vi "peakFinding dataSmooth.vi"(5 "Window":dbl=1.0 min=1.0 max=100000.0, 7 "Type":u8=1 min=1, 10 "dt":dbl=1.0, 11 "rawData":cluster{"xData":dbl[], "yData":dbl[]}) -> (3 "yData":dbl[](array[numeric]))   [LabVIEW 2018]
uses:
  PublicSubVI/Class/Sig2MS/Sig2MS.lvclass
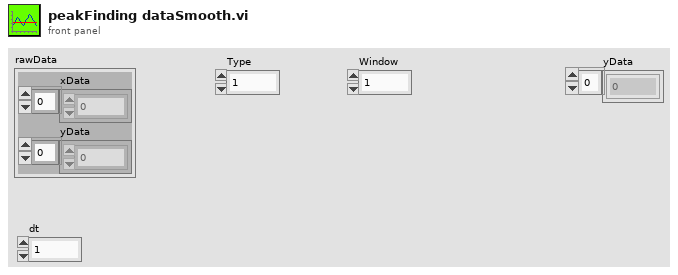
[diagram p1: front panel]
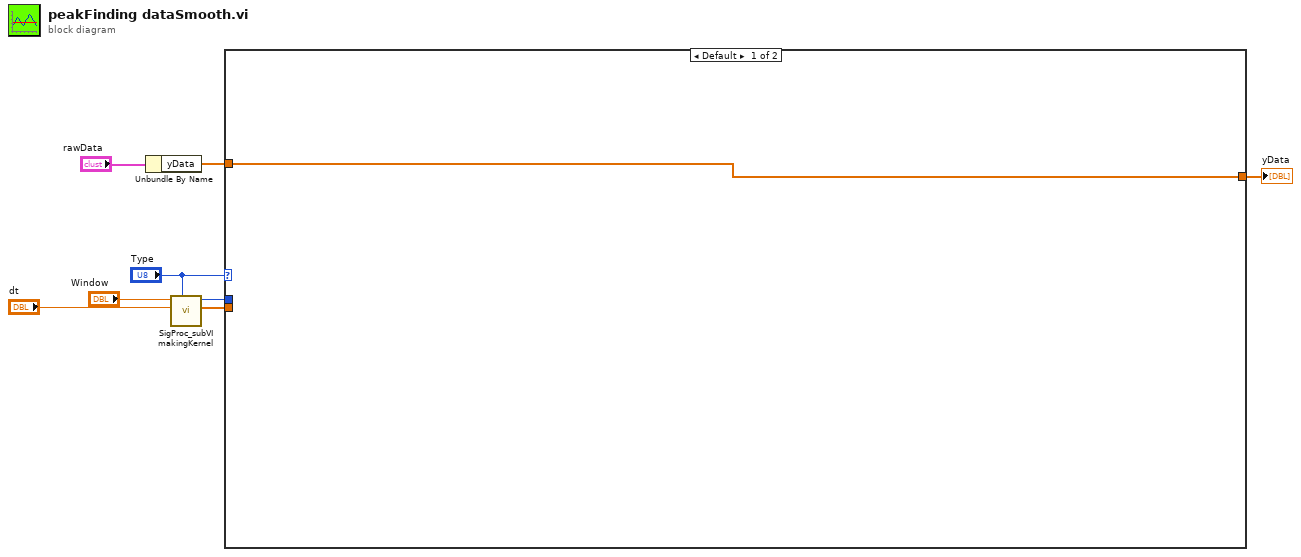
[diagram p0: block diagram]
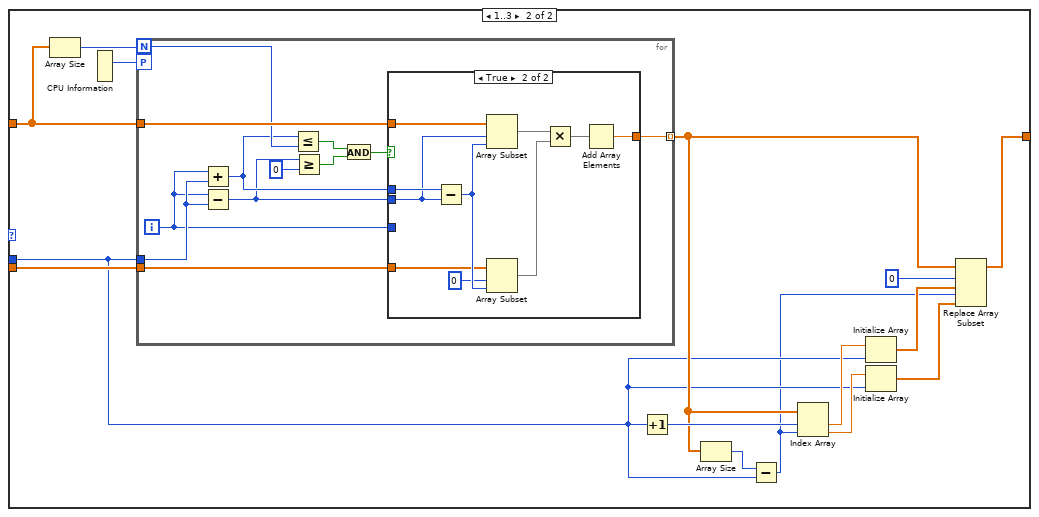
[diagram p2: hidden frame]
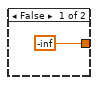
[diagram p3: hidden frame]
diagram:
  n1 = Unbundle By Name("rawData") -> ("yData"=w4:dbl[])
  n2 = call "SigProc_subVI makingKernel.vi"("Type"="Type", "dt"="dt", "Window"="Window") -> ("kernel"=w1:sgl[], "window"=w7:i32)  [unwired: 6 in, 1 out]
  n3 = case shown="Default" "Type" {
    tunnel: [w9 w11] -> w2
    tunnel: w4 -> [w9 w22]
    tunnel: w7 -> [_ w16]
    tunnel: w1 -> [_ w21]
    frame Default {
    }
    frame 1..3 {
      n4 = Array Size(array=w22) -> (size(s)=w23:i32)
      n5 = CPU Information() -> (5:w24:i32)  [unwired: 3 out]
      n6 = for {
        N: w23 -> [w31]
        workers-P: w24 -> [_]
        tunnel: [w36] -> w19 mode=indexing
        tunnel: w22 -> [w35]
        tunnel: w16 -> [w34]
        tunnel: w21 -> [w33]
        i -> [w26]
        n7 = Add(x=w26, y=w34) -> (x+y=w28:i32)
        n8 = Subtract(x=w26, y=w34) -> (x-y=w27:i32)
        n9 = Less Or Equal?(x=w28, y=w31) -> (x <= y?=w30:bool)
        n10 = Greater Or Equal?(x=w27, y=0) -> (x >= y?=w29:bool)
        n11 = And(x=w30, y=w29) -> (x .and. y?=w25:bool)
        n12 = case shown="True" w25 {
          tunnel: [-inf w43] -> w36
          tunnel: w35 -> [_ w42]
          tunnel: w33 -> [_ w40]
          tunnel: w28 -> [_ w39]
          tunnel: w27 -> [_ w38]
          tunnel: w26 -> [_ _]
          frame False {
          }
          frame True {
            n13 = Subtract(x=w39, y=w38) -> (x-y=w47:i32)
            n14 = Array Subset(array=w42, index=w38, length=w47) -> (w41:dbl[])
            n15 = Array Subset(array=w40, index=0, length=w47) -> (w45:sgl[])
            n16 = Multiply(x=w41, y=w45) -> (x*y=w44:dbl[])
            n17 = Add Array Elements(numeric array=w44) -> (sum=w43:dbl)
          }
        }
      }
      n18 = Increment(x=w16) -> (x+1=w20:i32)
      n19 = Array Size(array=w19) -> (size(s)=w13:i32)
      n20 = Subtract(x=w13, y=w16) -> (x-y=w10:i32)
      n21 = Index Array(array=w19, index #1=w20, index #2=w10) -> (element #1=w18:dbl, element #2=w17:dbl)
      n22 = Initialize Array(w18, w16) -> (w14:dbl[])
      n23 = Initialize Array(w17, w16) -> (w12:dbl[])
      n24 = Replace Array Subset(array=w19, new element #1=w14, index #1=0 ("index"), new element #2=w12, index #2=w10) -> (w11:dbl[])
    }
  }
  "yData" <- w2
